vi "Initialize.vi"(7 "Process ID":string, 8 "error in (no error)":errorcluster, 11 "Output Process in":refnum<class "Output Process.lvclass">) -> (0 "error out":errorcluster, 3 "Output Process out":refnum<class "Output Process.lvclass">)   [LabVIEW 2019, in "TelemetryAsync Engine.lvlib" / "Output Process.lvclass"]
uses:
  Output Process.lvclass
  Parent Classes/Process/Process.lvclass
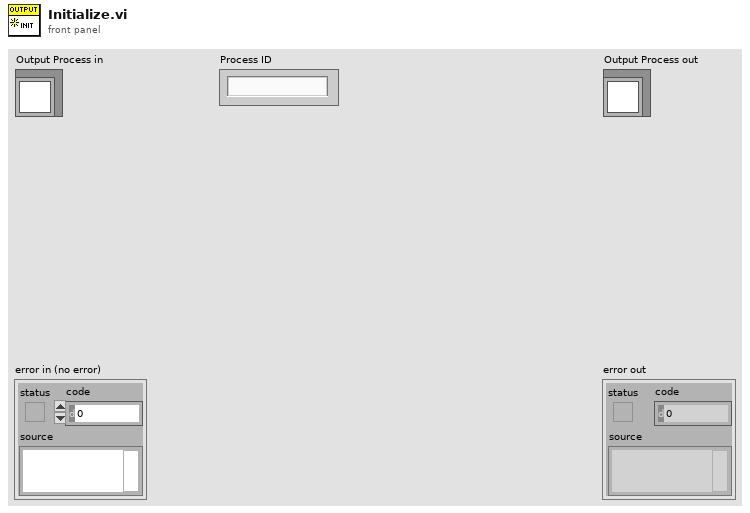
[diagram p1: front panel]
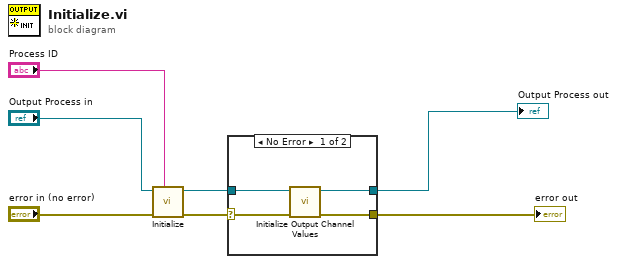
[diagram p0: block diagram]
diagram:
  n1 = call-parent "Initialize.vi"("Process ID"="Process ID", "error in (no error)"="error in (no error)", "Process in"="Output Process in") -> ("error out"=w4:errorcluster, "Process out"=w3:refnum<class "Output Process.lvclass">)  [unwired: 7 in]
  n2 = case shown="No Error" w4 {
    selector: w4 -> [w10 w12]
    tunnel: w3 -> [w11 w13]
    tunnel: [w9 w12] -> w2
    tunnel: [w8 w13] -> w1
    frame No Error {
      n3 = call "Initialize Output Channel Values.vi"("error in (no error)"=w10, "Output Process in"=w11) -> ("error out"=w9:errorcluster, "Output Process out"=w8:refnum<class "Output Process.lvclass">)  [unwired: 8 in]
    }
    frame Error {
    }
  }
  "error out" <- w2
  "Output Process out" <- w1
